vi "Msg.Event.Unregister.vi"(8 "Error (in)":errorcluster, 11 "Msg.Refs":T1) -> (0 "Error (out)":errorcluster)   [LabVIEW 2023, in "MessagingModule.lvlib"]
doc: "Used to unregister a user event."
uses:
  MessagingModule.lvlib
  Msg.Data.ctl
  Msg.Event.Ref.ctl
  Msg.Event.RegRef.ctl
  Msg.Q.Ref.ctl
  Msg.Noti.Ref.ctl
  Msg.Refs.ctl
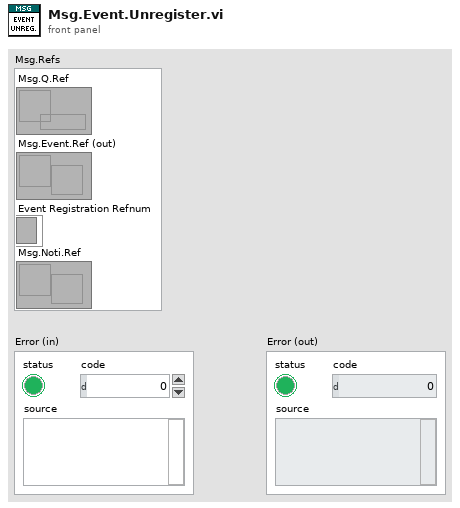
[diagram p1: front panel]
types:
  T1 = typedef "MessagingModule.lvlib/Msg.Refs.ctl" = cluster{"Msg.Q.Ref":T2, "Msg.Event.Ref (out)":T3, "Event Registration Refnum":T4, "Msg.Noti.Ref":T5}
  T2 = typedef "MessagingModule.lvlib/Msg.Q.Ref.ctl" = refnum<queue>
  T3 = typedef "MessagingModule.lvlib/Msg.Event.Ref.ctl" = refnum<user-event>
  T4 = typedef "MessagingModule.lvlib/Msg.Event.RegRef.ctl" = refnum<event-registration>
  T5 = typedef "MessagingModule.lvlib/Msg.Noti.Ref.ctl" = refnum<notifier>
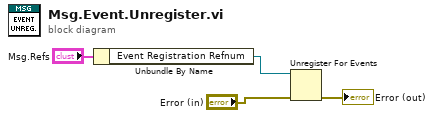
[diagram p0: block diagram]
diagram:
  n1 = Unbundle By Name("Msg.Refs") -> ("Event Registration Refnum"=w1:T4)
  n2 = Unregister For Events(event registration refnum=w1, error in="Error (in)") -> (error out=→"Error (out)":errorcluster)
